vi "task1_day2.vi"() -> ()   [LabVIEW 2017]
panel:
  out "Numeric":i32
  out "after substring":string
  out "length":i32
  in  "file path (use dialog)":path
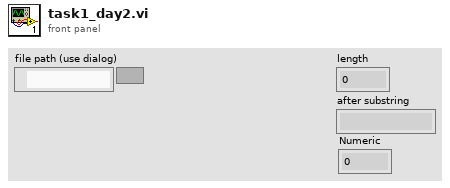
[diagram p1: front panel]
types:
  T1 = enum16{"open", "replace", "create", "open or create", "replace or create", "replace or create with confirmation"}
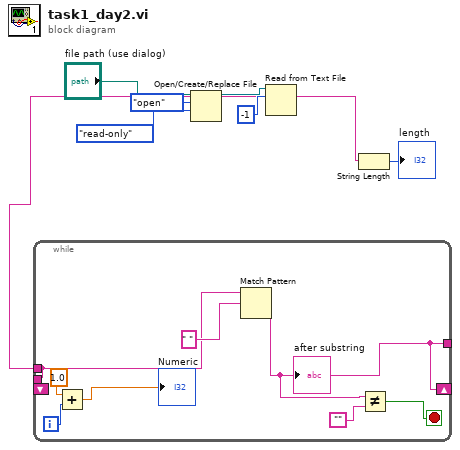
[diagram p0: block diagram]
diagram:
  n1 = Open/Create/Replace File(file path (use dialog)="file path (use dialog)", operation (0:open)=T1."open", access (0:read/write)=enum16{"read/write", "read-only", "write-only"}."read-only") -> (refnum out=w4:refnum<file>)  [unwired: 3 in, 2 out]
  n2 = Read from Text File(file (use dialog)=w4, count=-1) -> (text=w2:string)  [unwired: 2 in, 3 out]
  n3 = while {
    tunnel: w2 -> [w10]
    tunnel: [w9] -> _
    shift-right: [w9] -> _
    shift-left: w1 -> [_]
    tunnel: [w10] -> w1
    i -> [w11]
    stop <- w14 stop-if-true
    n4 = Add(x=1.0, y=w11) -> (x+y=→"Numeric":dbl)
    n5 = Match Pattern(string=w10, regular expression=" ") -> (after substring=w9:string)  [unwired: 1 in, 3 out]
    "after substring" <- w9
    n6 = Not Equal?(x=w9, y="") -> (x != y?=w14:bool)
  }
  n7 = String Length(string=w2) -> (length=→"length":i32)
